vi "Raft_wars_Ver6.vi"() -> ()   [LabVIEW 2026]
panel:
  out "Computer Board":dbl[][](array[numeric])
  out "Player  Board":dbl[][](array[numeric])
  in  "Player Ship Inputs":T1(array[cluster]) {"Y-Coordinate" min=0 max=7; "X-Coordinate" min=0 max=7}
  in  "Emergency Stop":bool
  out "Game Status":string
  out "Ships Placed":dbl
  out "Losses":dbl
  out "Computer Hits":dbl
  out "Wins":dbl
  out "Player Hits":dbl
  in  "Attack":bool
  in  "Play Again":bool
  in  "Place Ship":bool
  in  "Attack Y":dbl
  in  "Attack X":dbl
  in  "Ship Y":i32
  in  "Ship X":i32
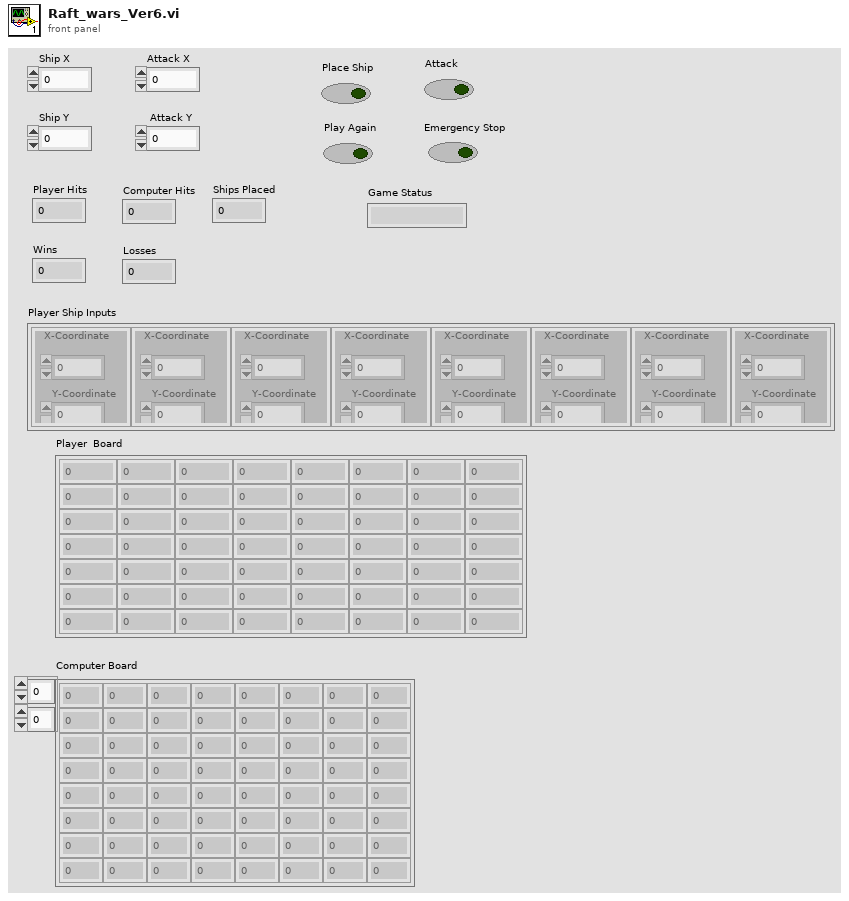
[diagram p1: front panel]
types:
  T1 = cluster{"X-Coordinate":i32, "Y-Coordinate":i32}[]
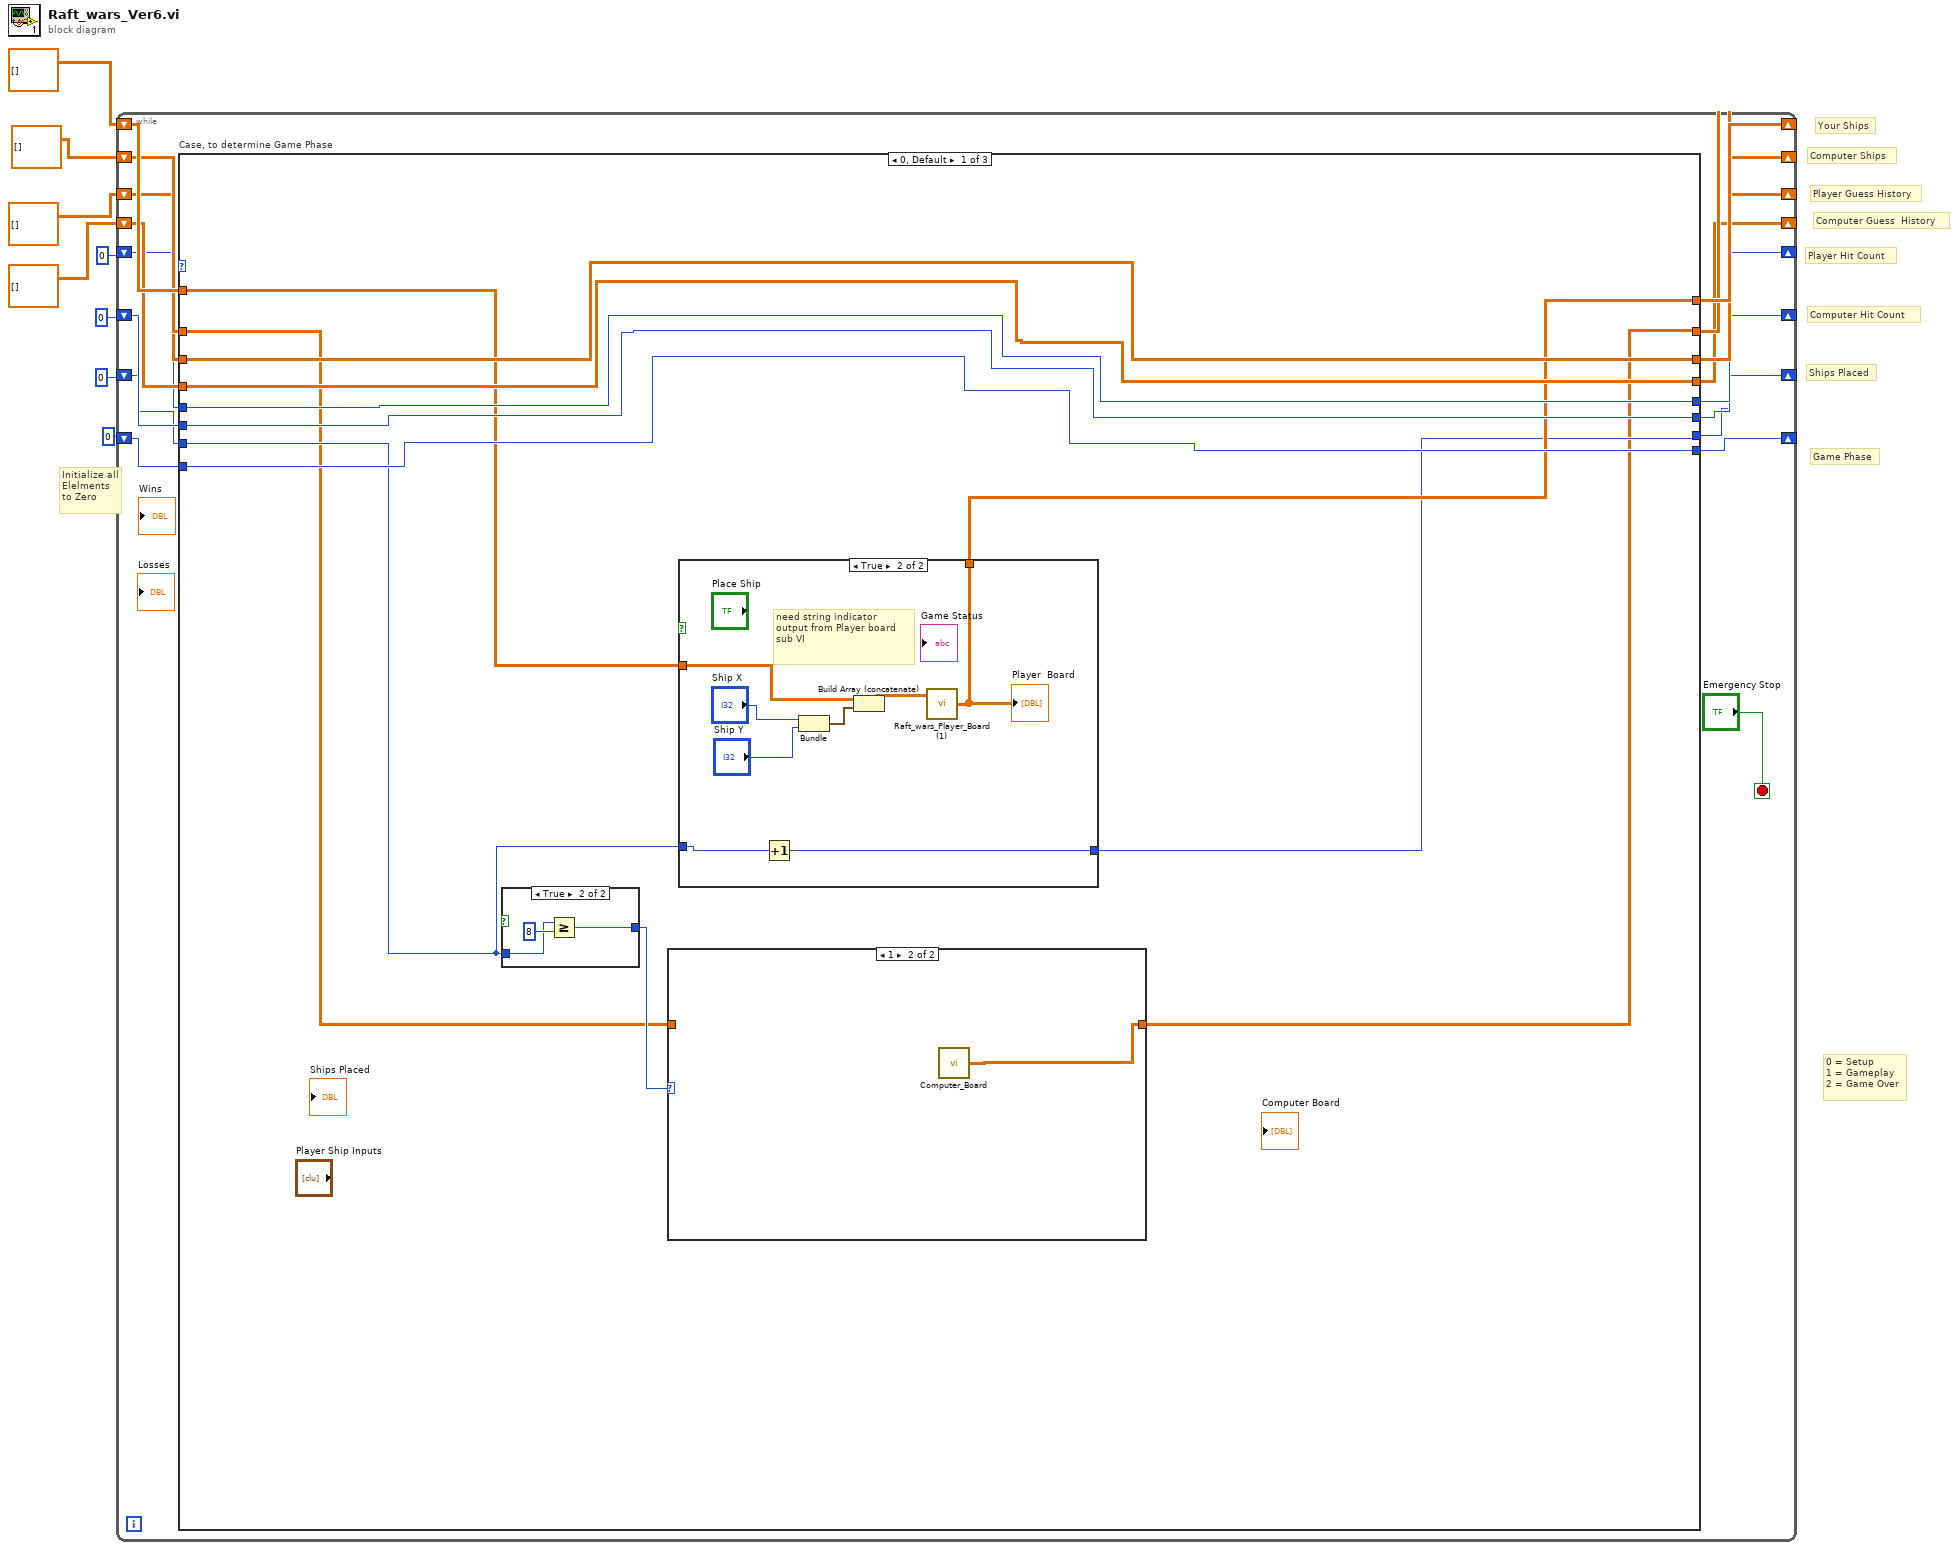
[diagram p0: block diagram]
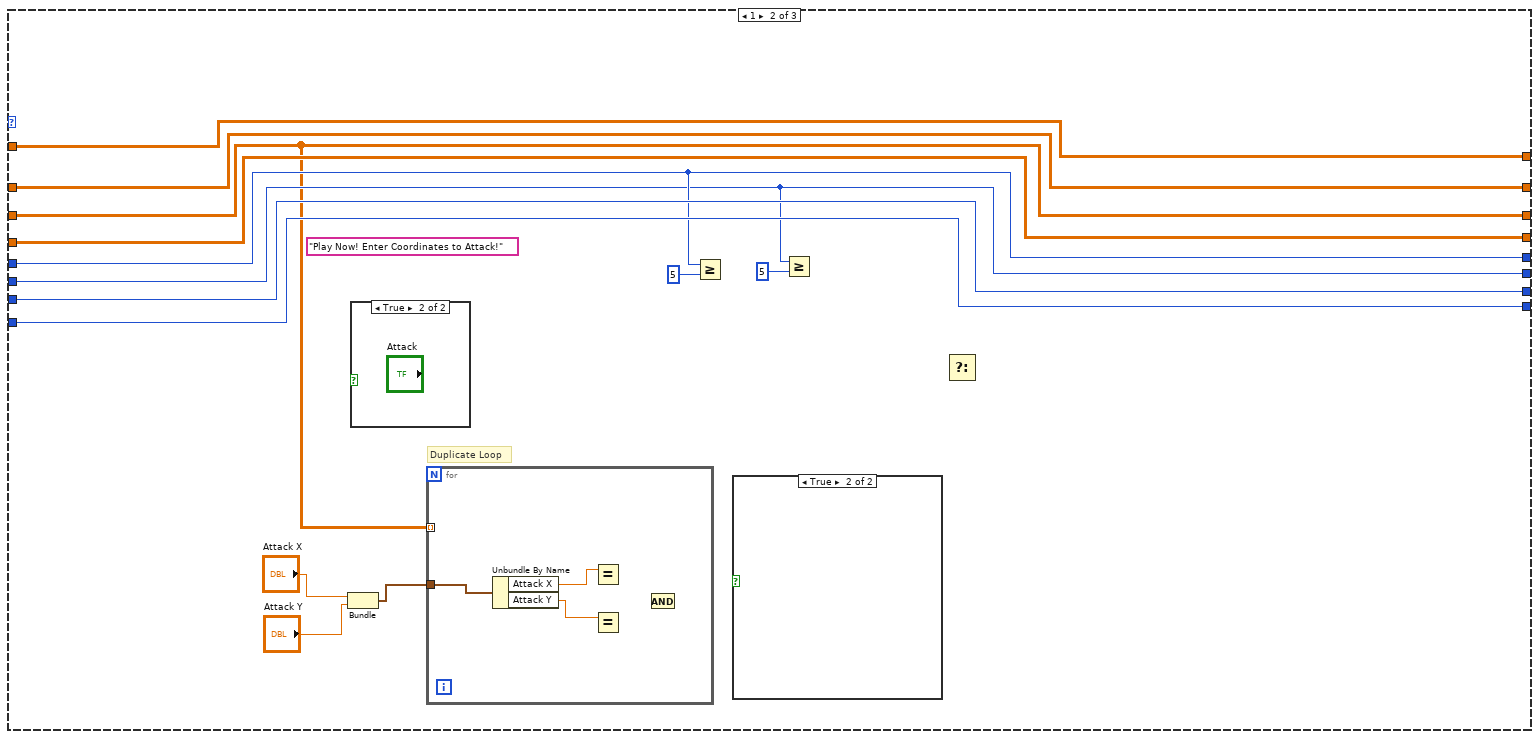
[diagram p5: hidden frame]
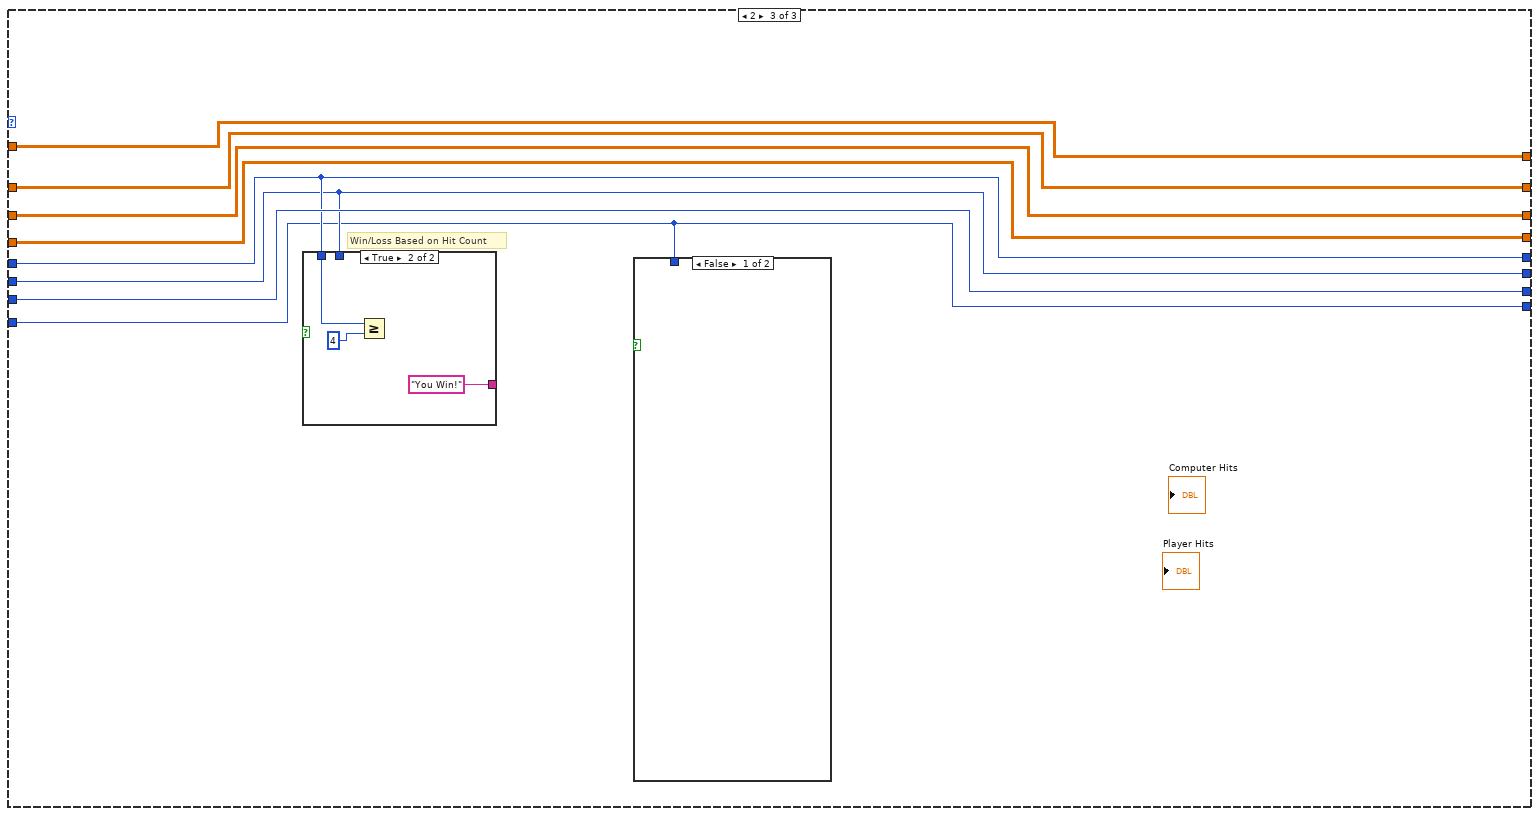
[diagram p8: hidden frame]
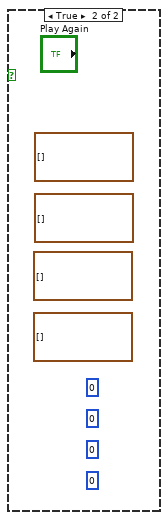
[diagram p9: hidden frame]
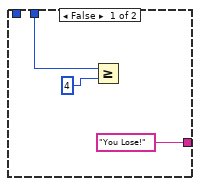
[diagram p10: hidden frame]
diagram:
  # "0 = Setup\n1 = Gameplay\n2 = Game Over"
  # "Initialize all\nElelments\nto Zero"
  # "Ships Placed"
  # "Your Ships"
  # "Computer Ships"
  # "Player Guess History"
  # "Computer Guess  History"
  # "Player Hit Count"
  # "Computer Hit Count"
  # "Game Phase"
  n1 = while {
    shift-right: [w23] -> _
    shift-left: dbl[][] [] ("Array") -> [w24]
    shift-right: [w21] -> _
    shift-left: dbl[][] [] ("Array") -> [w22]
    shift-right: [w19] -> _
    shift-left: dbl[][] [] ("Array") -> [w20]
    shift-right: [w17] -> _
    shift-left: dbl[][] [] ("Array") -> [w18]
    shift-right: [w12] -> _
    shift-left: 0 -> [w16]
    shift-right: [w11] -> _
    shift-left: 0 -> [w15]
    shift-right: [w10] -> _
    shift-left: 0 -> [w14]
    shift-right: [w9] -> _
    shift-left: 0 -> [w13]
    stop <- "Emergency Stop" stop-if-true
    n2 = case "Case, to determine Game Phase" shown="0, Default" {
      selector: _ -> [_ _ _]
      tunnel: w24 -> [w32 w66 w77]
      tunnel: [w30 w66 w77] -> w23
      tunnel: w22 -> [w27 w58 w76]
      tunnel: [w26 w58 w76] -> w21
      tunnel: w20 -> [w37 w54 w75]
      tunnel: [w37 w54 w75] -> w19
      tunnel: w18 -> [w36 w65 w74]
      tunnel: [w36 w65 w74] -> w17
      tunnel: w16 -> [w35 w61 w72]
      tunnel: w15 -> [w34 w59 w71]
      tunnel: w14 -> [w31 w64 w73]
      tunnel: w13 -> [w33 w63 w70]
      tunnel: [w35 w61 w72] -> w12
      tunnel: [w34 w59 w71] -> w11
      tunnel: [w29 w64 w73] -> w10
      tunnel: [w33 w63 w70] -> w9
      frame 0, Default {
        n3 = case shown="True" {
          selector: _ -> [_ _]
          tunnel: w31 -> [w40 w42]
          tunnel: [w40 w41] -> w28
          frame False {
          }
          frame True {
            n4 = Greater Or Equal?(x=w42, y=8) -> (x >= y?=w41:bool)
          }
        }
        n5 = case shown="1" w28 {
          tunnel: w27 -> [w38 _]
          tunnel: [w38 w39] -> w26
          frame 0, Default {
          }
          frame 1 {
            n6 = call "Computer_Board.vi"() -> ("Array"=w39:dbl[][])
          }
        }
        n7 = case shown="True" {
          selector: _ -> [_ _]
          tunnel: w32 -> [w45 w49]
          tunnel: w31 -> [w44 w48]
          tunnel: [w45 w47] -> w30
          tunnel: [w44 w46] -> w29
          frame False {
          }
          frame True {
            # "need string indicator\noutput from Player board \nsub VI"
            n8 = Increment(x=w48) -> (x+1=w46:i32)
            n9 = Bundle("Ship X"="Ship X", "Ship Y"="Ship Y") -> (w51:cluster{"Ship X":i32, "Ship Y":i32})  [unwired: 1 in]
            n10 = Build Array (concatenate)(w49, w51) -> (w50:dbl[][])
            n11 = call "Raft_wars_Player_Board (1).vi"("Player Ship Inputs"=w50) -> ("Array"=w47:dbl[][])
            "Player  Board" <- w47
          }
        }
      }
      frame 1 {
        (unwired) "Play Now! Enter Coordinates to Attack!"
        # "Duplicate Loop"
        n12 = Bundle("Attack X"="Attack X", "Attack Y"="Attack Y") -> (w55:cluster{"Attack X":dbl, " Attack Y":dbl})  [unwired: 1 in]
        n13 = case shown="True" {
          selector: _ -> [_ _]
          frame False {
          }
          frame True {
          }
        }
        n14 = for {
          tunnel: w55 -> [w69]
          tunnel: w54 -> [_] mode=indexing
          n15 = Unbundle By Name(w69) -> ("Attack X"=w68:dbl, "Attack Y"=w67:dbl)
          n16 = Equal?(x=w68) -> ()  [unwired: 1 in, 1 out]
          n17 = Equal?(x=w67) -> ()  [unwired: 1 in, 1 out]
          n18 = And() -> ()  [unwired: 2 in, 1 out]
        }
        n19 = Greater Or Equal?(x=w61, y=5) -> ()  [unwired: 1 out]
        n20 = case shown="True" {
          selector: _ -> [_ _]
          frame False {
          }
          frame True {
          }
        }
        n21 = Greater Or Equal?(x=w59, y=5) -> ()  [unwired: 1 out]
        n22 = Select() -> ()  [unwired: 3 in, 1 out]
      }
      frame 2 {
        # "Win/Loss Based on Hit Count"
        n23 = case shown="True" {
          selector: _ -> [_ _]
          tunnel: w72 -> [_ w83]
          tunnel: ["You Lose!" "You Win!"] -> _
          tunnel: w71 -> [w78 _]
          frame False {
            n24 = Greater Or Equal?(x=w78, y=4) -> ()  [unwired: 1 out]
          }
          frame True {
            n25 = Greater Or Equal?(x=w83, y=4) -> ()  [unwired: 1 out]
          }
        }
        n26 = case shown="False" {
          selector: _ -> [_ _]
          tunnel: w70 -> [_ _]
          frame False {
          }
          frame True {
            (unwired) 0
            (unwired) 0
            (unwired) 0
            (unwired) cluster{dbl, dbl}[] []
            (unwired) cluster{dbl, dbl}[] []
            (unwired) cluster{dbl, dbl}[] []
            (unwired) cluster{dbl, dbl}[] []
            (unwired) 0
          }
        }
      }
    }
  }
